vi "image_arrays_to_difference_map.vi"(7 "normalize":bool=TRUE, 9 "capt_images":u8[][][](array[numeric]), 11 "orig_pattern":u8[][][](array[numeric])) -> (2 "dbl_diff_map":dbl[][](array[numeric]))   [LabVIEW 2011]
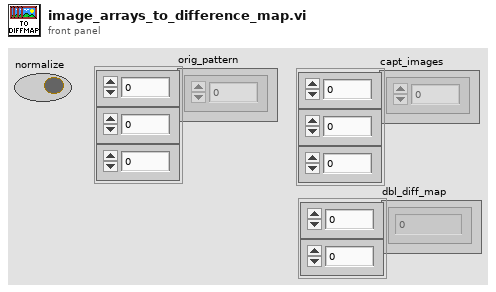
[diagram p1: front panel]
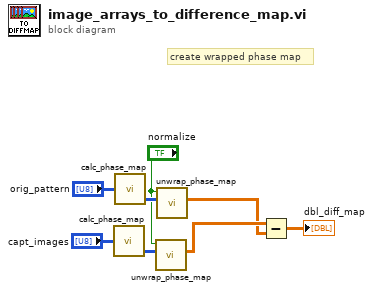
[diagram p0: block diagram]
diagram:
  # "create wrapped phase map"
  n1 = call "calc_phase_map.vi"("u8_ar_image_pixel_array"="capt_images") -> ("raw phase map array"=w6:u8[][])  [unwired: 3 in, 1 out]
  n2 = call "calc_phase_map.vi"("u8_ar_image_pixel_array"="orig_pattern") -> ("raw phase map array"=w5:u8[][])  [unwired: 3 in, 1 out]
  n3 = call "unwrap_phase_map.vi"("u8_ar_phase map"=w6, "normalize (y)"="normalize") -> ("df_ar_unwrapped_px_ar"=w3:dbl[][])  [unwired: 8 in, 1 out]
  n4 = call "unwrap_phase_map.vi"("u8_ar_phase map"=w5, "normalize (y)"="normalize") -> ("df_ar_unwrapped_px_ar"=w2:dbl[][])  [unwired: 8 in, 1 out]
  n5 = Subtract(x=w3, y=w2) -> (x-y=→"dbl_diff_map":dbl[][])
